vi "Filter Modifier.vi"(11 "Button Cluster 1":T1) -> (3 "Button Cluster Out":T1)   [LabVIEW 2014]
uses:
  Button Cluster.ctl
  Common Code/Change Detect Boolean.vi
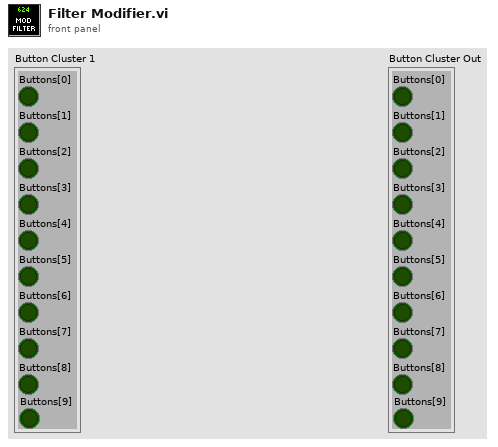
[diagram p1: front panel]
types:
  T1 = typedef "Button Cluster.ctl" = cluster{"Buttons[0]":bool, "Buttons[1]":bool, "Buttons[2]":bool, "Buttons[3]":bool, "Buttons[4]":bool, "Buttons[5]":bool, "Buttons[6]":bool, "Buttons[7]":bool, "Buttons[8]":bool, "Buttons[9]":bool}
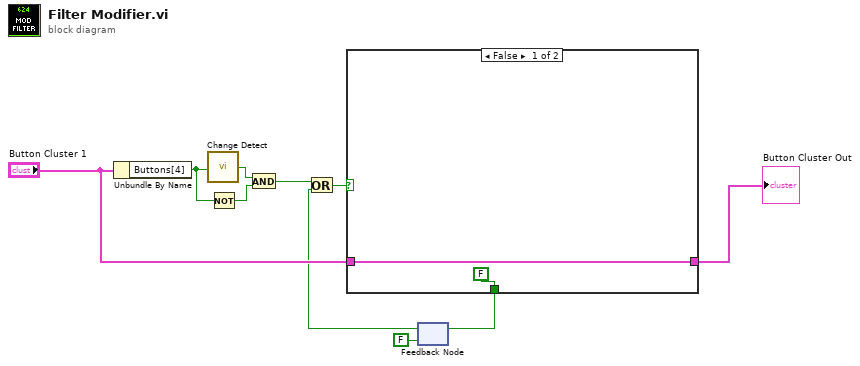
[diagram p0: block diagram]
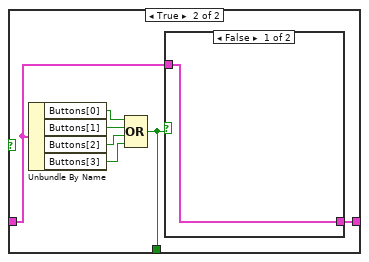
[diagram p2: hidden frame]
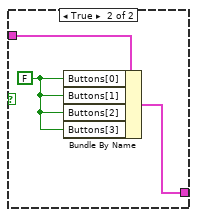
[diagram p3: hidden frame]
diagram:
  n1 = Unbundle By Name("Button Cluster 1") -> ("Buttons[4]"=w9:bool)
  n2 = call-poly "Change Detect.vi"("In"=w9) -> ("Changed?"=w10:bool)
  n3 = Not(x=w9) -> (.not. x?=w8:bool)
  n4 = And(x=w10, y=w8) -> (x .and. y?=w4:bool)
  n5 = feedback #1(FALSE) -> (w2:bool)
  n6 = Or(x=w4, y=w2) -> (x .or. y?=w3:bool)
  n7 = case shown="False" w3 {
    tunnel: "Button Cluster 1" -> [w12 w15]
    tunnel: [w12 w14] -> w6
    tunnel: [FALSE w13] -> w5
    frame False {
    }
    frame True {
      n8 = Unbundle By Name(w15) -> ("Buttons[0]"=w19:bool, "Buttons[1]"=w18:bool, "Buttons[2]"=w17:bool, "Buttons[3]"=w16:bool)
      n9 = Compound Arithmetic op=OR(w19, w18, w17, w16) -> (w13:bool)
      n10 = case shown="False" w13 {
        tunnel: w15 -> [w20 w23]
        tunnel: [w20 w21] -> w14
        frame False {
        }
        frame True {
          w22 = FALSE ("Buttons[0]")
          n11 = Bundle By Name(cluster=w23, "Buttons[0]"=w22, "Buttons[1]"=w22, "Buttons[2]"=w22, "Buttons[3]"=w22) -> (w21:T1)
        }
      }
    }
  }
  "Button Cluster Out" <- w6
  n12 = feedback-in #1(w5) -> ()
